vi "Collision Detection top level.vi"(0 "Model rotation (absolute, degrees)":sgl, 1 "Model rotation axis (unit vector)":sgl[](array[numeric])=[0.0, 0.0, 1.0], 3 "Model rotation axis coordinates (absolute, mm)":sgl[](array[numeric])=[0.0, 0.0, 0.0], 4 "Collision mode":T1=enum."Traverse - All", 5 "Get minimum separation within look-out sphere":bool, 6 "Traverse position (absolute, mm)":sgl[](array[numeric])=[0.0, 0.0, 0.0], 7 "3D graphics output":bool, 9 "Visualisation only (no collision detection)":bool, 10 "Traverse name":string, 11 "Extrusion mode":bool, 12 "Rig geometry directory path":path, 13 "Traverse extruded position":sgl[](array[numeric])=[0.0, 0.0, 0.0]) -> (14 "Collision":bool, 15 "Collision point(s)":sgl[][](array[numeric]), 17 "Minimum separation":sgl, 18 "Minimum separation vector (from trav.)":sgl[](array[numeric]), 19 "Error out":errorcluster)   [LabVIEW 2014]
uses:
  Collision Mode.ctl
  Typedefs/Triangle.ctl
  <vilib>/Utility/miscctls.llb/LVRGBAColorTypeDef.ctl
  Collision Detection global.vi
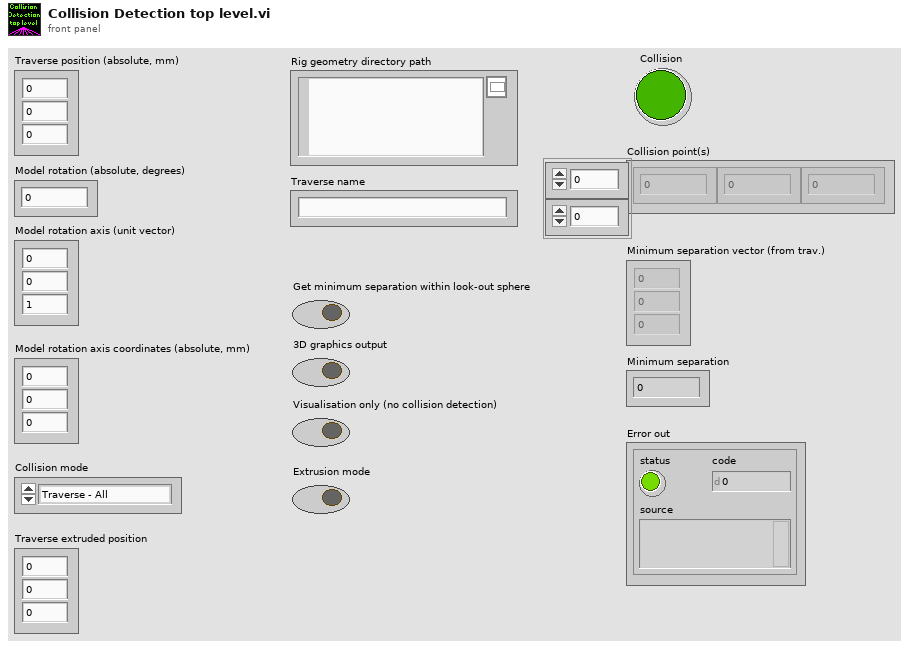
[diagram p1: front panel]
types:
  T1 = typedef "Collision Mode.ctl" = enum16{"Traverse - Tunnel", "Traverse - Model", "Traverse - Traverse", "Traverse - All"}
  T2 = typedef "LVRGBAColorTypeDef.ctl" = cluster{"Red":sgl, "Green":sgl, "Blue":sgl, "Alpha":sgl}
  T3 = cluster{"Red":sgl, "Green":sgl, "Blue":sgl, "Alpha":sgl}
  T4 = typedef "TreeNodeBox.ctl" = cluster{"Face 0":T5, "Face 1":T5, "Face 2":T5, "Face 3":T5, "Face 4":T5, "Face 5":T5, "Level":i32, "Pmax":sgl[], "Pmin":sgl[], "Parent":i32, "Child 1":i32, "Child 2":i32, "Child 3":i32, "Child 4":i32, "Child 5":i32, "Child 6":i32, "Child 7":i32, "Child 8":i32, "Triangles":i32[], "is leaf node":bool}
  T5 = typedef "Quad.ctl" = cluster{"V0":sgl[], "V1":sgl[], "V2":sgl[], "V3":sgl[], "E0":sgl[], "E1":sgl[], "E2":sgl[], "E3":sgl[], "n^":sgl[], "nE0^":sgl[], "nE1^":sgl[], "nE2^":sgl[], "nE3^":sgl[]}
  T6 = typedef "Triangle.ctl" = cluster{"V0":sgl[], "V1":sgl[], "V2":sgl[], "E0":sgl[], "E1":sgl[], "E2":sgl[], "n^":sgl[], "nE0^":sgl[], "nE1^":sgl[], "nE2^":sgl[]}
  T7 = typedef "Sphere.ctl" = cluster{"Centre":sgl[], "Radius":sgl}
  T8 = enum16{"Inherit Value", "Points", "Wireframe", "Polygons"}
  T9 = typedef "LV3DPointTypeDef.ctl" = cluster{"X":sgl, "Y":sgl, "Z":sgl}
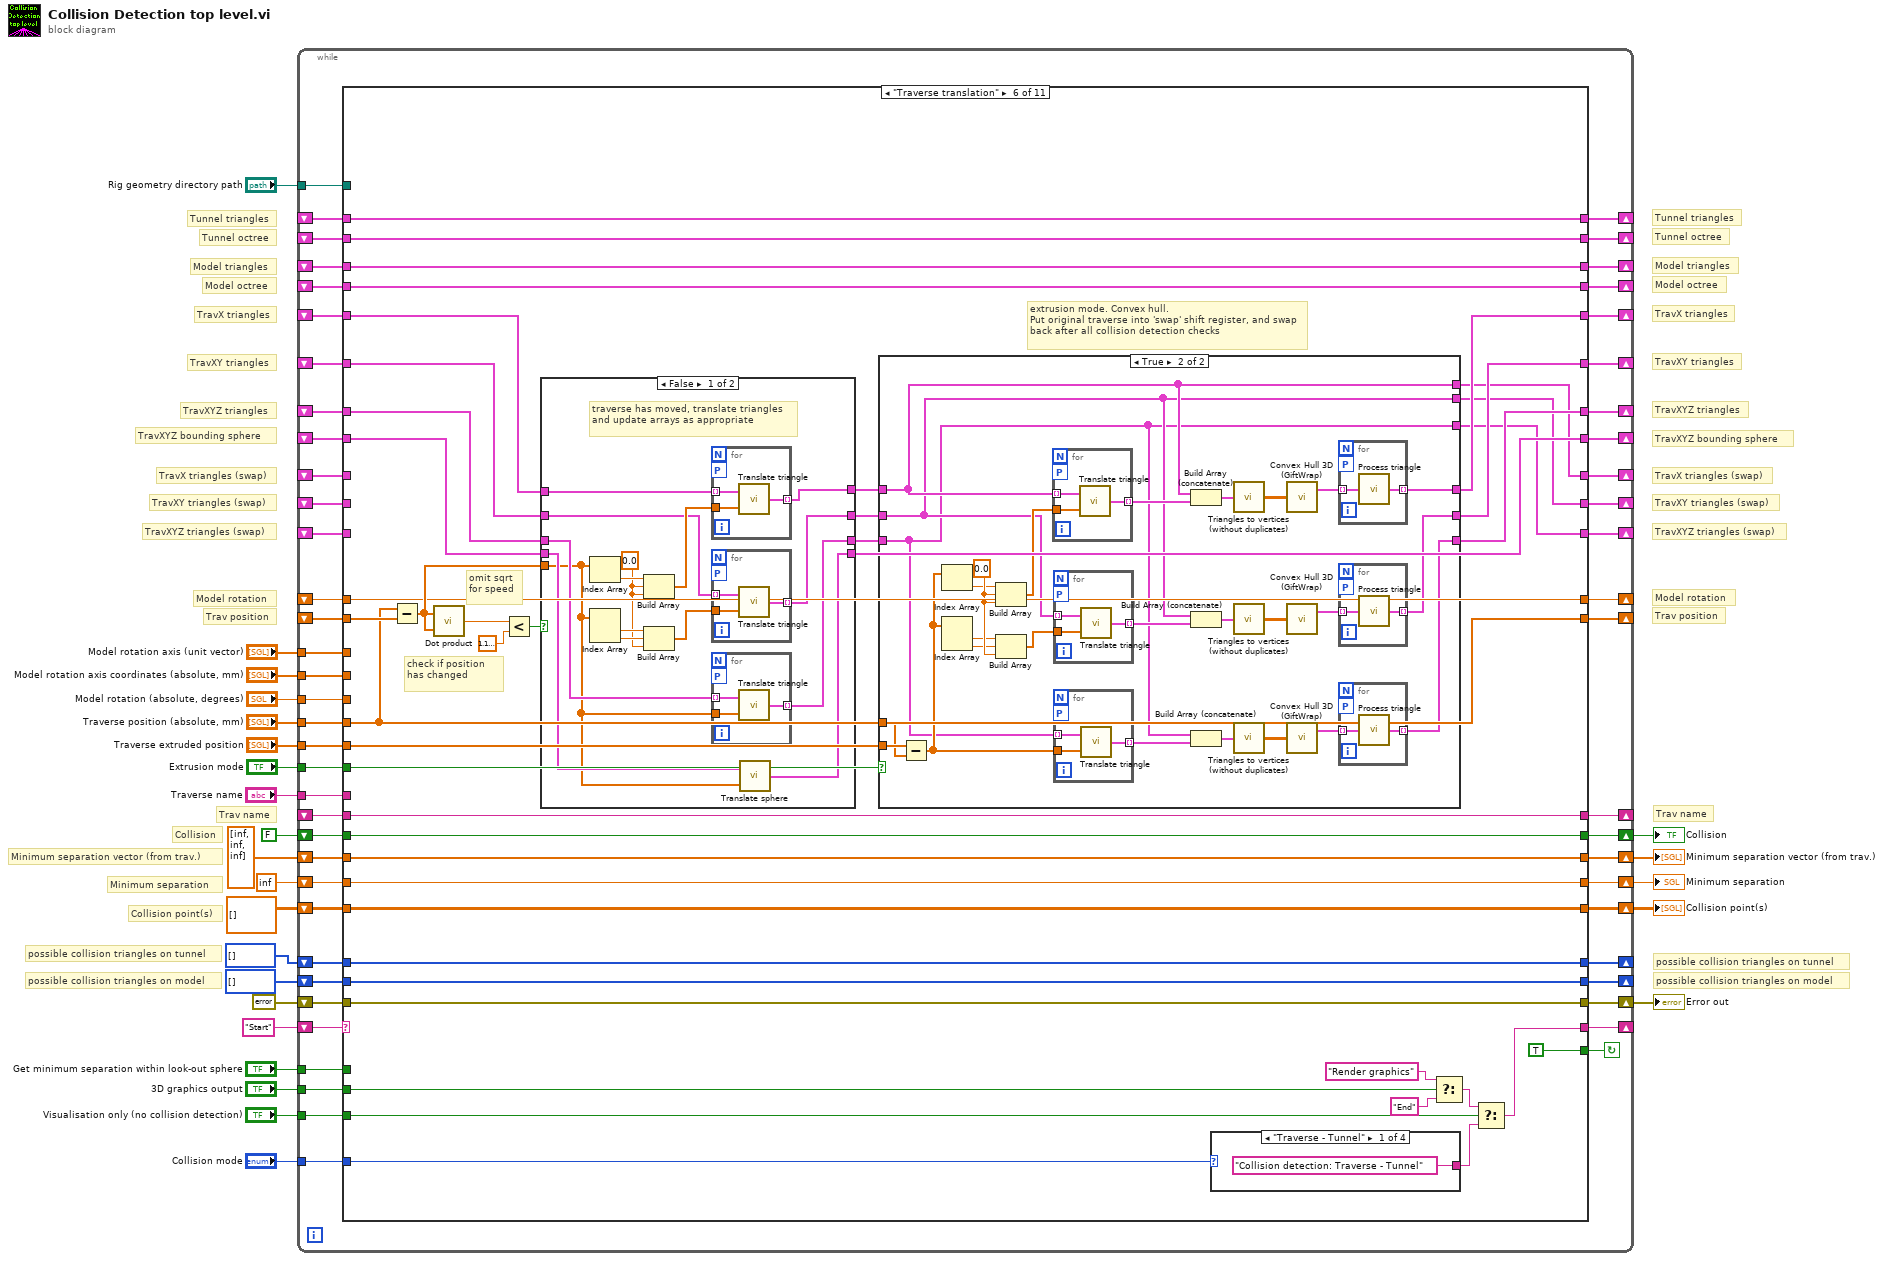
[diagram p0: block diagram]
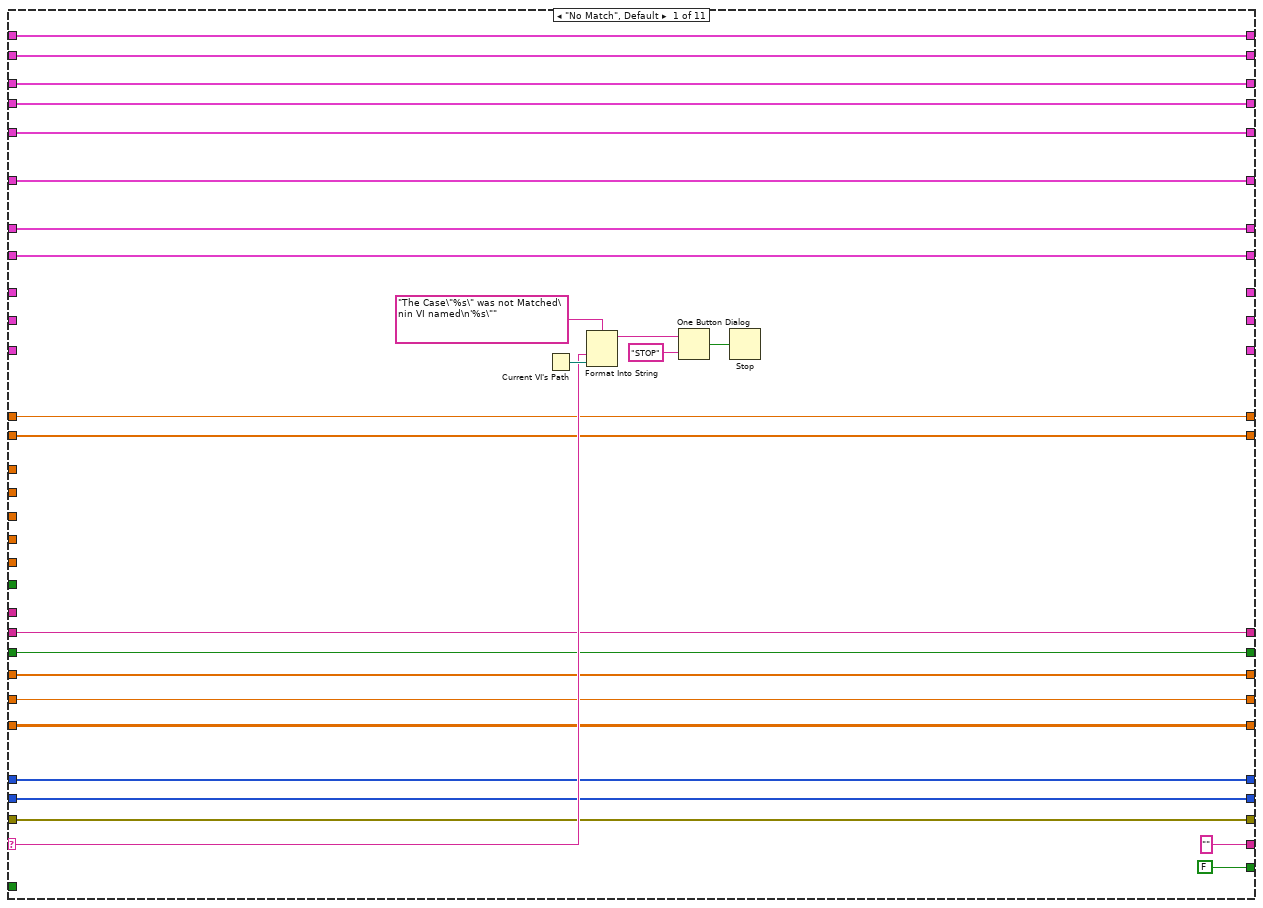
[diagram p2: hidden frame]
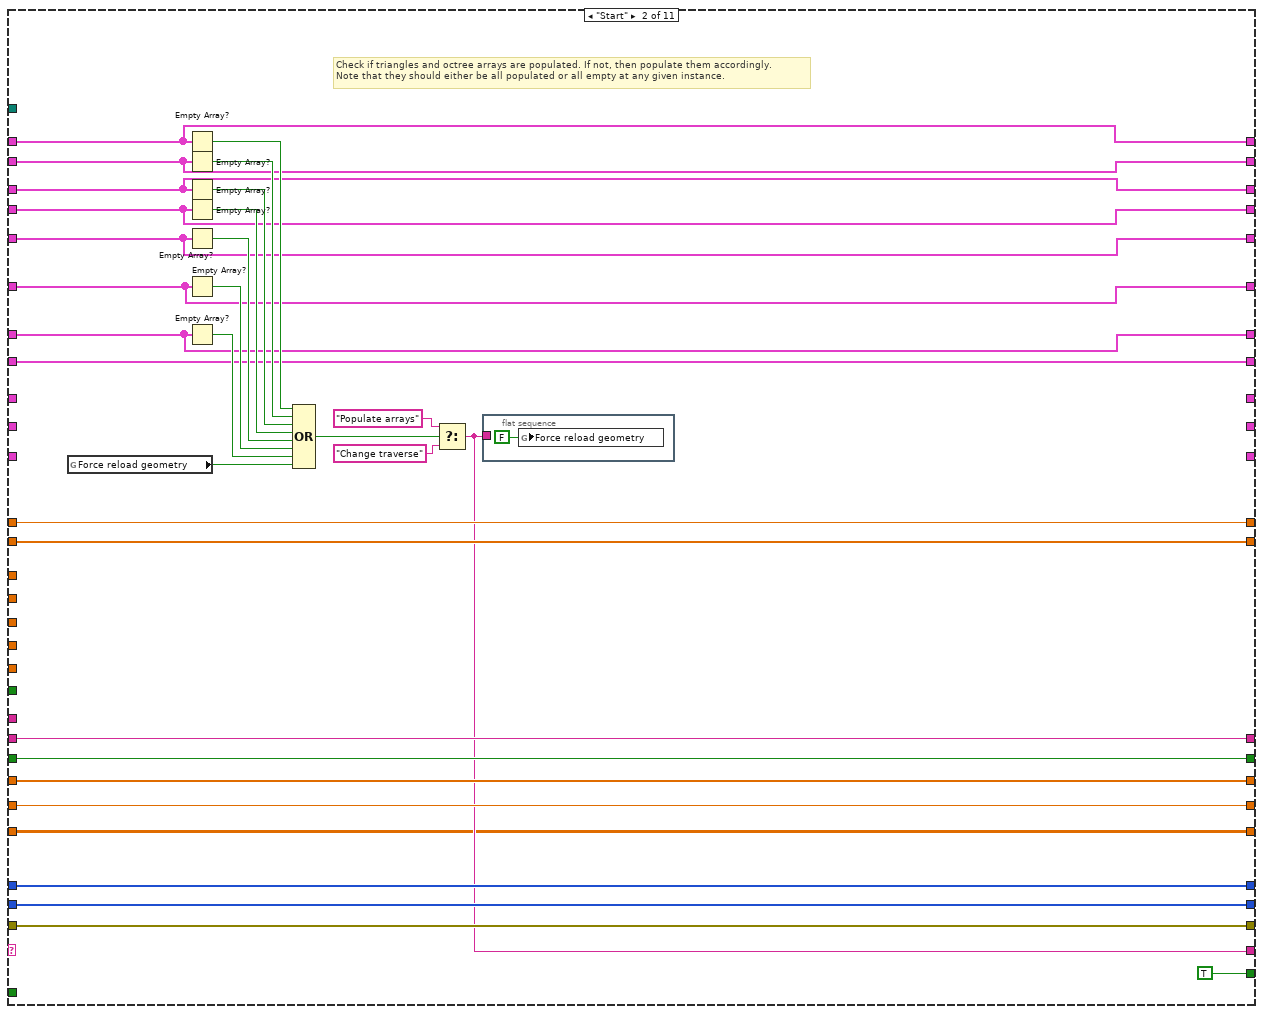
[diagram p3: hidden frame]
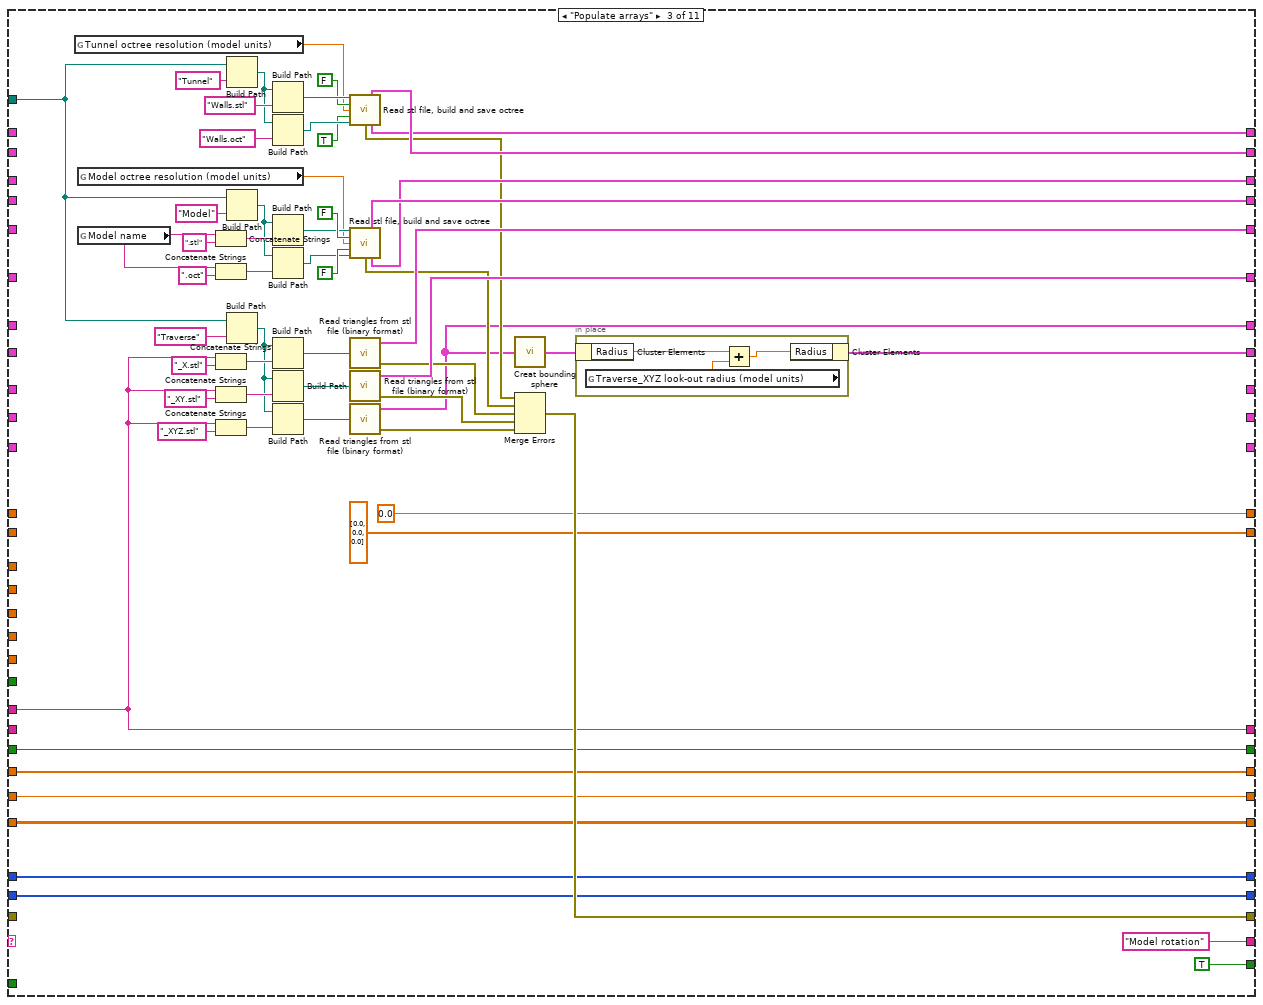
[diagram p4: hidden frame]
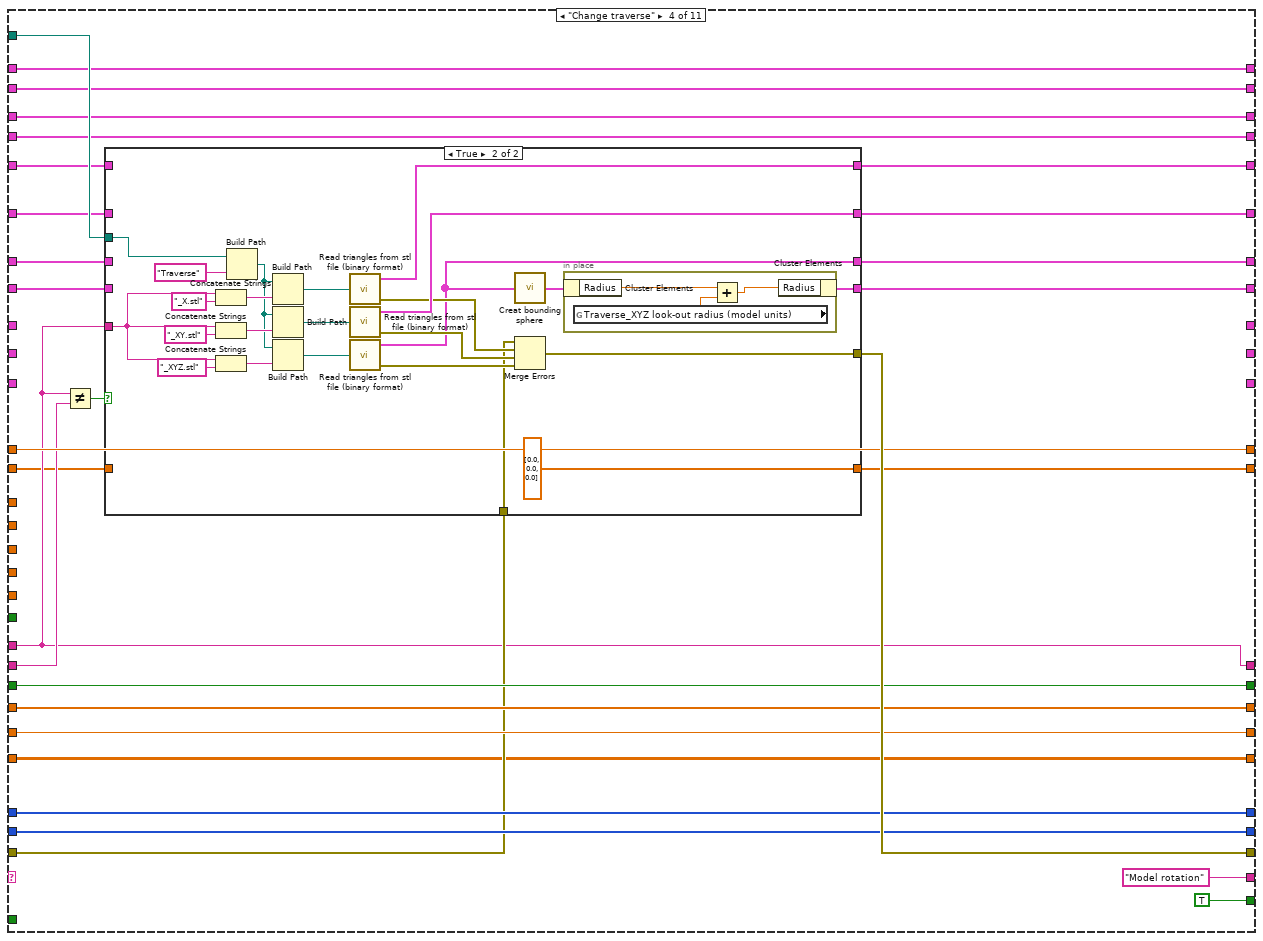
[diagram p5: hidden frame]
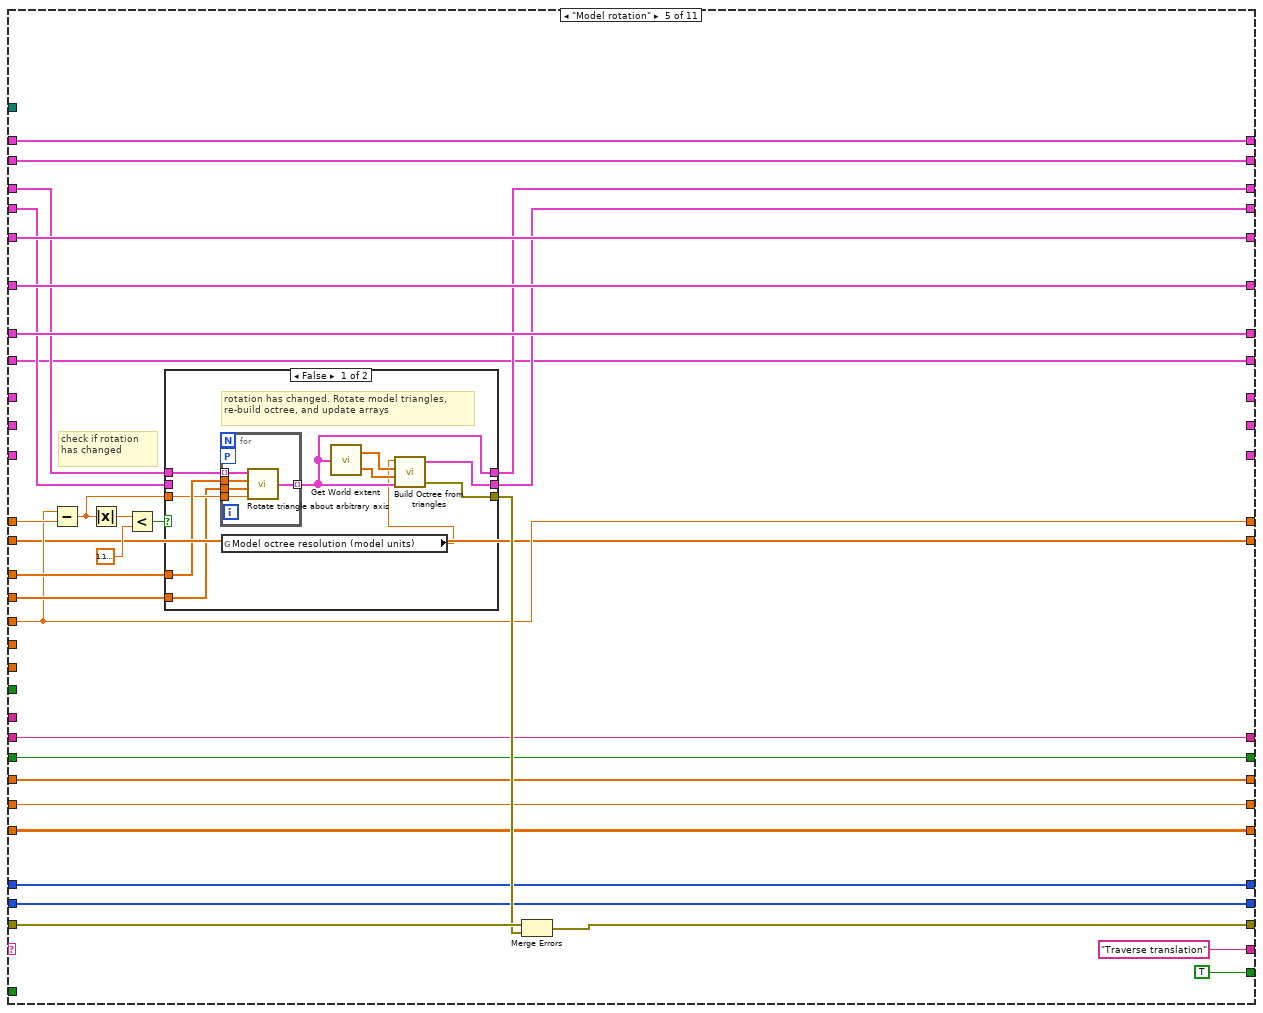
[diagram p7: hidden frame]
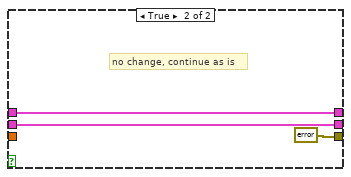
[diagram p8: hidden frame]
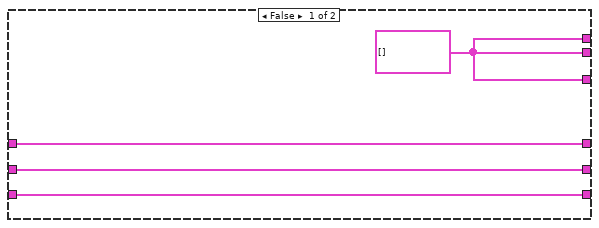
[diagram p9: hidden frame]
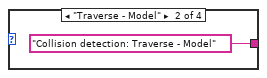
[diagram p10: hidden frame]
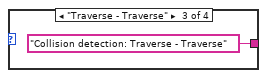
[diagram p11: hidden frame]
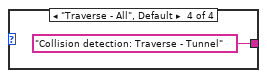
[diagram p12: hidden frame]
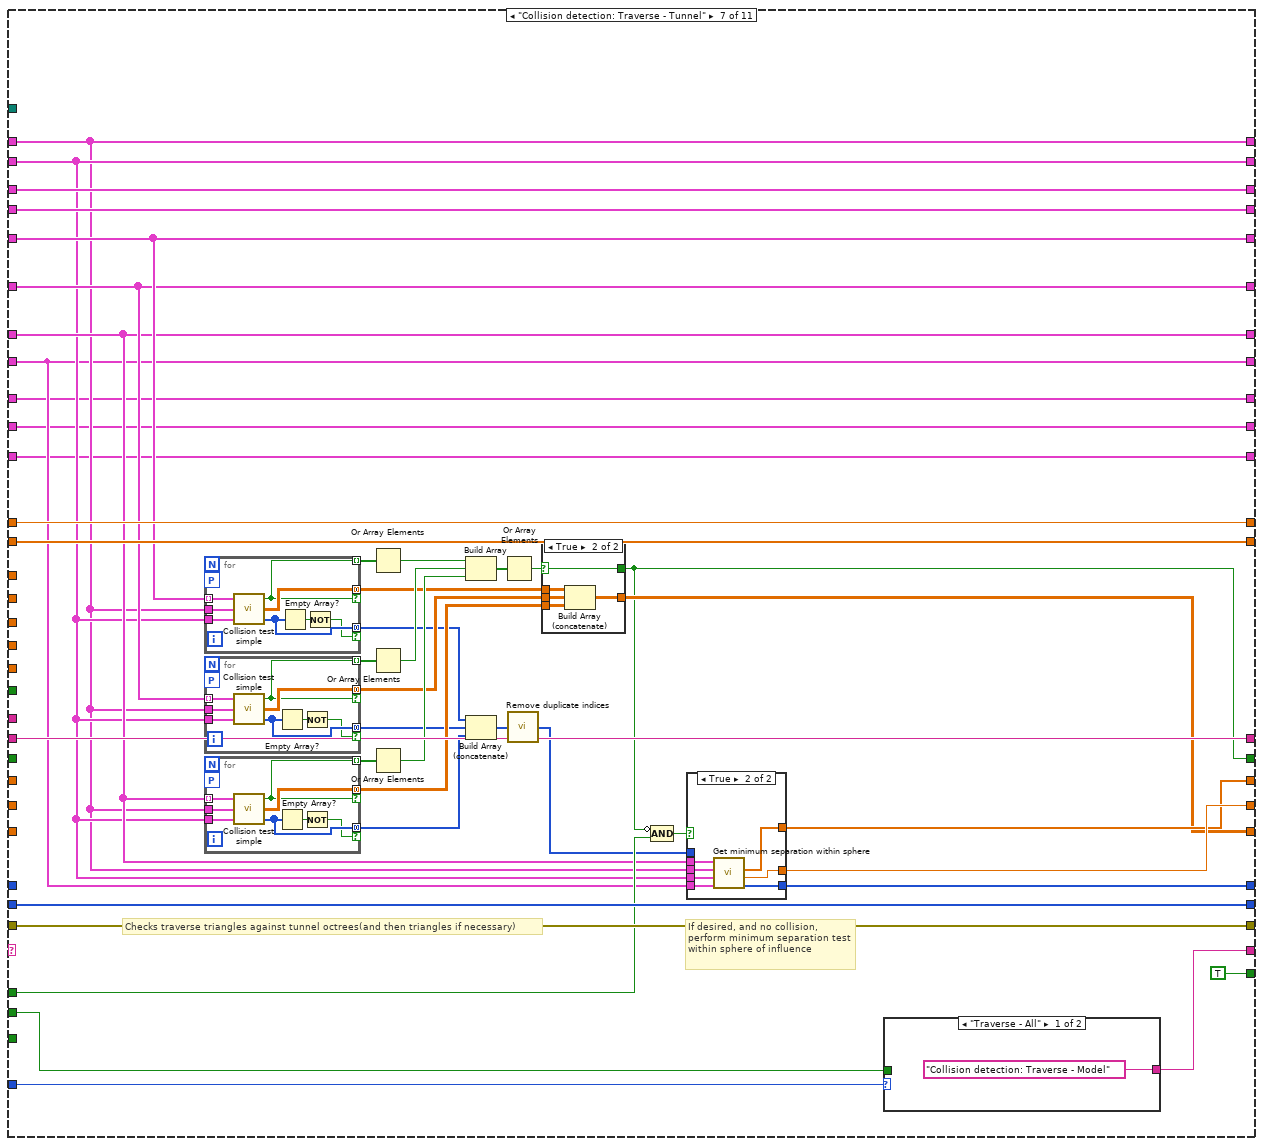
[diagram p14: hidden frame]
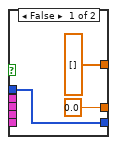
[diagram p15: hidden frame]
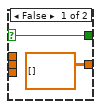
[diagram p16: hidden frame]
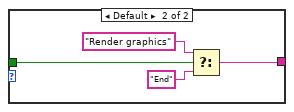
[diagram p17: hidden frame]
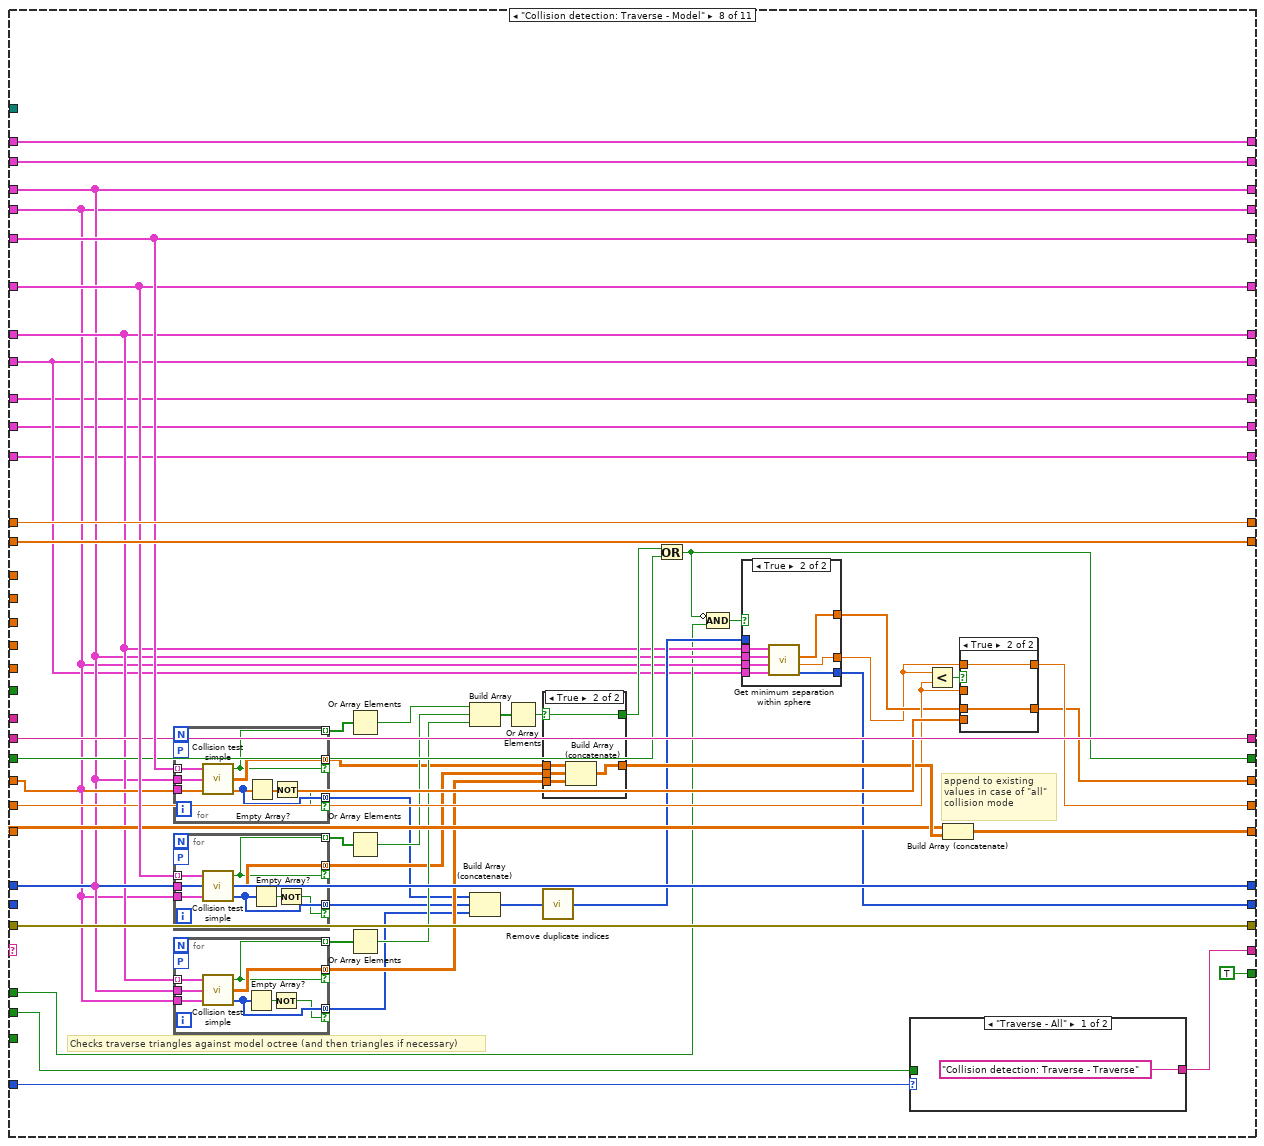
[diagram p18: hidden frame]
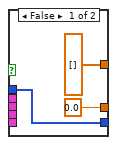
[diagram p19: hidden frame]
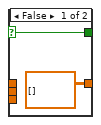
[diagram p20: hidden frame]
diagram:
  # "TravXYZ triangles (swap)"
  # "TravXY triangles (swap)"
  # "TravX triangles (swap)"
  # "TravXYZ triangles (swap)"
  # "TravXY triangles (swap)"
  # "TravX triangles (swap)"
  # "TravXYZ bounding sphere"
  # "TravXYZ bounding sphere"
  # "Trav name"
  # "Collision"
  # "Minimum separation vector (from trav.)"
  # "Minimum separation"
  # "Collision point(s)"
  # "Trav name"
  # "possible collision triangles on tunnel"
  # "possible collision triangles on model"
  # "possible collision triangles on tunnel"
  # "possible collision triangles on model"
  # "Model rotation"
  # "Trav position"
  # "TravXYZ triangles"
  # "TravXY triangles"
  # "TravX triangles"
  # "Model octree"
  # "Model triangles"
  # "Tunnel octree"
  # "Tunnel triangles"
  # "Model rotation"
  # "Trav position"
  # "TravXYZ triangles"
  # "TravXY triangles"
  # "TravX triangles"
  # "Model octree"
  # "Model triangles"
  # "Tunnel octree"
  # "Tunnel triangles"
  n1 = while {
    shift-right: [w64] -> _
    shift-left: "Start" -> [w82]
    shift-right: [w71] -> _
    shift-left: _ -> [w81]
    shift-right: [w70] -> _
    shift-left: _ -> [w80]
    shift-right: [w69] -> _
    shift-left: _ -> [w79]
    shift-right: [w68] -> _
    shift-left: _ -> [w78]
    shift-right: [w67] -> _
    shift-left: _ -> [w77]
    shift-right: [w66] -> _
    shift-left: _ -> [w76]
    shift-right: [w65] -> _
    shift-left: _ -> [w54]
    shift-right: [w58] -> _
    shift-left: _ -> [w74]
    shift-right: [w57] -> _
    shift-left: _ -> [w75]
    tunnel: "Traverse position (absolute, mm)" -> [w72]
    tunnel: "Model rotation (absolute, degrees)" -> [w73]
    tunnel: "Rig geometry directory path" -> [w62]
    shift-right: [w60] -> w12
    shift-left: errorcluster {"status"=FALSE, "code"=0, "source"=""} ("error IO") -> [w59]
    tunnel: "Model rotation axis (unit vector)" -> [w56]
    tunnel: "Model rotation axis coordinates (absolute, mm)" -> [w55]
    tunnel: "Get minimum separation within look-out sphere" -> [w53]
    tunnel: "Visualisation only (no collision detection)" -> [w52]
    tunnel: "3D graphics output" -> [w51]
    shift-right: [w47] -> _
    shift-left: i32[] [] ("I32 array without duplicates") -> [w45]
    shift-right: [w46] -> _
    shift-left: i32[] [] ("I32 array without duplicates") -> [w44]
    shift-right: [w48] -> w14
    shift-left: sgl[] [inf, inf, inf] -> [w43]
    shift-right: [w49] -> w15
    shift-left: sgl inf -> [w42]
    shift-right: [w36] -> w13
    shift-left: sgl[][] [] -> [w41]
    shift-right: [w50] -> w16
    shift-left: FALSE -> [w40]
    shift-right: [w39] -> _
    shift-left: _ -> [w61]
    tunnel: "Traverse name" -> [w38]
    tunnel: "Collision mode" -> [w37]
    shift-right: [w34] -> _
    shift-left: _ -> [w35]
    tunnel: "Traverse extruded position" -> [w33]
    tunnel: "Extrusion mode" -> [w32]
    shift-right: [w31] -> _
    shift-left: _ -> [w28]
    shift-right: [w30] -> _
    shift-left: _ -> [w27]
    shift-right: [w29] -> _
    shift-left: _ -> [w26]
    stop <- w63 continue-if-true
    n2 = case shown="\"Traverse translation\"" w82 {
      selector: w82 -> [w103 _ _ _ _ _ _ _ _ _ _]
      tunnel: w81 -> [w99 w121 _ w218 w291 w350 w440 w571 w643 w710 w825]
      tunnel: w80 -> [w98 w122 _ w217 w290 w349 w441 w570 w642 w706 w824]
      tunnel: w79 -> [w97 w123 _ w216 w286 w348 w472 w531 w639 w666 w823]
      tunnel: w78 -> [w96 w124 _ w215 w279 w347 w471 w530 w638 w705 w822]
      tunnel: w77 -> [w95 w125 _ w211 w289 w354 w474 w572 w644 w709 w804]
      tunnel: w76 -> [w94 w126 _ w210 w288 w353 w473 w569 w641 w708 w805]
      tunnel: w54 -> [w93 w127 _ w209 w287 w352 w442 w532 w640 w707 w806]
      tunnel: w75 -> [w91 w119 _ w207 w267 w357 w477 w575 w651 w714 w827]
      tunnel: w74 -> [w92 w120 _ w224 w284 w331 w478 w576 w652 w715 w826]
      tunnel: w73 -> [_ _ _ _ w274 _ _ _ _ _ _]
      tunnel: w72 -> [_ _ _ _ _ w323 _ _ _ _ _]
      tunnel: [w99 w121 w194 w218 w291 w350 w440 w571 w643 w710 w825] -> w71
      tunnel: [w98 w122 w195 w217 w290 w349 w441 w570 w642 w706 w824] -> w70
      tunnel: [w97 w123 w196 w216 w281 w348 w472 w531 w639 w666 w823] -> w69
      tunnel: [w96 w124 w197 w215 w280 w347 w471 w530 w638 w705 w822] -> w68
      tunnel: [w95 w125 w198 w229 w289 w319 w474 w572 w644 w709 w809] -> w67
      tunnel: [w94 w126 w199 w230 w288 w318 w473 w569 w641 w708 w808] -> w66
      tunnel: [w93 w127 w143 w231 w287 w317 w442 w532 w640 w707 w807] -> w65
      tunnel: [w92 w120 sgl 0.0 ("Numeric") w224 w274 w331 w478 w576 w652 w715 w826] -> w58
      tunnel: [w91 w119 sgl[] [0.0, 0.0, 0.0] ("Traverse position (absolute, mm)") w206 w267 w323 w477 w575 w651 w714 w827] -> w57
      tunnel: w62 -> [_ _ w193 w228 _ _ _ _ _ _ _]
      tunnel: ["" w111 "Model rotation" "Model rotation" "Traverse translation" w343 w463 w560 w647 "End" "" ("f")] -> w64
      tunnel: [FALSE TRUE TRUE TRUE TRUE TRUE TRUE TRUE TRUE TRUE FALSE] -> w63
      tunnel: w61 -> [w85 w113 _ w213 w268 w333 w468 w568 w637 w675 w816]
      tunnel: [w100 w128 w192 w227 w278 w345 w475 w573 w645 w693 w828] -> w60
      tunnel: w59 -> [w100 w128 _ w214 w277 w345 w475 w573 w645 w694 w828]
      tunnel: w56 -> [_ _ _ _ w292 _ _ _ _ _ _]
      tunnel: w55 -> [_ _ _ _ w282 _ _ _ _ _ _]
      tunnel: w53 -> [_ _ _ _ _ _ w446 w529 _ _ _]
      tunnel: w52 -> [_ _ _ _ _ w344 _ _ _ _ _]
      tunnel: w51 -> [_ _ _ _ _ w342 w464 w559 w648 _ _]
      tunnel: [w86 w114 w152 w219 w269 w334 w447 w533 w636 w711 w817] -> w50
      tunnel: [w87 w115 w153 w220 w270 w335 w470 w564 w634 w712 w818] -> w49
      tunnel: [w88 w116 w154 w221 w271 w336 w469 w563 w635 w713 w819] -> w48
      tunnel: [w84 w110 w144 w205 w266 w328 w466 w566 w631 w658 w815] -> w36
      tunnel: [w90 w117 w155 w222 w272 w337 w443 w567 w633 w685 w820] -> w47
      tunnel: [w89 w118 w156 w223 w273 w338 w467 w534 w632 w664 w821] -> w46
      tunnel: w45 -> [w90 w117 w155 w222 w272 w337 _ w567 w633 w685 w820]
      tunnel: w44 -> [w89 w118 w156 w223 w273 w338 w467 _ w632 w664 w821]
      tunnel: w43 -> [w88 w116 w154 w221 w271 w336 _ w562 w635 w713 w819]
      tunnel: w42 -> [w87 w115 w153 w220 w270 w335 _ w554 w634 w712 w818]
      tunnel: w41 -> [w84 w110 w144 w205 w266 w328 _ w555 w631 w658 w815]
      tunnel: w40 -> [w86 w114 w152 w219 w269 w334 _ w557 w636 w711 w817]
      tunnel: [w85 w113 w151 w208 w268 w333 w468 w568 w637 w675 w816] -> w39
      tunnel: w38 -> [_ _ w151 w208 _ _ _ _ _ _ _]
      tunnel: w37 -> [_ _ _ _ _ w330 w465 w561 _ _ _]
      tunnel: w35 -> [w83 w109 _ w203 w265 w327 w439 w528 w630 w657 w814]
      tunnel: [w83 w109 w141 w204 w265 w326 w439 w528 w630 w657 w814] -> w34
      tunnel: w33 -> [_ _ _ _ _ w324 _ _ _ _ _]
      tunnel: w32 -> [_ _ _ _ _ w325 _ _ _ _ w813]
      tunnel: [_ _ _ _ _ w314 w438 w527 w629 w656 _] -> w31
      tunnel: [_ _ _ _ _ w315 w437 w526 w628 w655 _] -> w30
      tunnel: [_ _ _ _ _ w316 w436 w525 w627 w654 _] -> w29
      tunnel: w28 -> [_ _ _ _ _ _ w438 w527 w629 w656 w812]
      tunnel: w27 -> [_ _ _ _ _ _ w437 w526 w628 w655 w811]
      tunnel: w26 -> [_ _ _ _ _ _ w436 w525 w627 w654 w810]
      frame "No Match", Default {
        n3 = Current VI's Path() -> (path=w104:path)
        n4 = Format Into String(format string="The Case\"%s\" was not Matched\nin VI named\n'%s\"" ("Format String"), w103, w104) -> (resulting string=w107:string)  [unwired: 2 in, 1 out]
        n5 = One Button Dialog(message=w107, button name ("OK")="STOP") -> (true=w105:bool)
        n6 = Stop(stop? (T)=w105) -> ()
      }
      frame "Start" {
        # "Check if triangles and octree arrays are populated. If not, then populate them accordingly.\nNote that they should either be all populated or all empty at any given instance."
        n7 = global read "Collision Detection global.vi" "Force reload geometry"() -> (w112:bool)
        n8 = Empty Array?(array=w121) -> (empty?=w139:bool)
        n9 = Empty Array?(array=w122) -> (empty?=w138:bool)
        n10 = Empty Array?(array=w123) -> (empty?=w137:bool)
        n11 = Empty Array?(array=w124) -> (empty?=w136:bool)
        n12 = Empty Array?(array=w125) -> (empty?=w135:bool)
        n13 = Empty Array?(array=w126) -> (empty?=w134:bool)
        n14 = Empty Array?(array=w127) -> (empty?=w133:bool)
        n15 = Compound Arithmetic op=OR(w139, w138, w137, w136, w135, w134, w133, w112) -> (w132:bool)
        n16 = Select(t="Populate arrays", s=w132, f="Change traverse") -> (s? t:f=w111:string)
        n17 = flat-sequence {
          tunnel: w111 -> [_]
          frame #0 {
            n18 = global write "Collision Detection global.vi" "Force reload geometry"(FALSE ("Force reload geometry")) -> ()
          }
        }
      }
      frame "Populate arrays" {
        n19 = global read "Collision Detection global.vi" "Tunnel octree resolution (model units)"() -> (w149:sgl)
        n20 = global read "Collision Detection global.vi" "Model octree resolution (model units)"() -> (w148:sgl)
        n21 = global read "Collision Detection global.vi" "Model name"() -> (w147:string)
        n22 = Concatenate Strings(w147, ".stl" ("string")) -> (w180:string)
        n23 = Concatenate Strings(w147, ".oct" ("string")) -> (w179:string)
        n24 = Concatenate Strings(w151, "_X.stl" ("string")) -> (w173:string)
        n25 = Concatenate Strings(w151, "_XY.stl" ("string")) -> (w164:string)
        n26 = Concatenate Strings(w151, "_XYZ.stl" ("string")) -> (w162:string)
        n27 = Build Path(base path=w193, name or relative path="Tunnel") -> (appended path=w188:path)
        n28 = Build Path(base path=w193, name or relative path="Model") -> (appended path=w178:path)
        n29 = Build Path(base path=w193, name or relative path="Traverse") -> (appended path=w150:path)
        n30 = Build Path(base path=w188, name or relative path="Walls.stl") -> (appended path=w189:path)
        n31 = Build Path(base path=w188, name or relative path="Walls.oct") -> (appended path=w186:path)
        n32 = Build Path(base path=w178, name or relative path=w180) -> (appended path=w175:path)
        n33 = Build Path(base path=w178, name or relative path=w179) -> (appended path=w174:path)
        n34 = Build Path(base path=w150, name or relative path=w173) -> (appended path=w170:path)
        n35 = Build Path(base path=w150, name or relative path=w164) -> (appended path=w166:path)
        n36 = Build Path(base path=w150, name or relative path=w162) -> (appended path=w160:path)
        n37 = call "Read stl file, build and save octree.vi"("STL file path (load)"=w189, "Auto resolution"=FALSE, "Specify resolution"=w149, "Invert model (interior region)"=TRUE, "Octree file path (save)"=w186) -> ("Octree node array"=w195:T4[], "Error out"=w169:errorcluster, "Triangles array"=w194:T6[])  [unwired: 3 in, 5 out]
        n38 = call "Read stl file, build and save octree.vi"("STL file path (load)"=w175, "Auto resolution"=FALSE, "Specify resolution"=w148, "Invert model (interior region)"=FALSE, "Octree file path (save)"=w174) -> ("Octree node array"=w197:T4[], "Error out"=w168:errorcluster, "Triangles array"=w196:T6[])  [unwired: 3 in, 5 out]
        n39 = call "Read triangles from stl file (binary format).vi"("STL file path"=w170) -> ("Triangles array"=w198:T6[], "Error out"=w167:errorcluster)  [unwired: 1 out]
        n40 = call "Read triangles from stl file (binary format).vi"("STL file path"=w166) -> ("Triangles array"=w199:T6[], "Error out"=w163:errorcluster)  [unwired: 1 out]
        n41 = call "Read triangles from stl file (binary format).vi"("STL file path"=w160) -> ("Triangles array"=w143:T6[], "Error out"=w159:errorcluster)  [unwired: 1 out]
        n42 = call "Creat bounding sphere.vi"("Triangles"=w143) -> ("Bounding sphere"=w142:T7)
        n43 = Merge Errors(w169, w168, w167, w163, w159) -> (w192:errorcluster)
        n44 = in-place {
          n45 = in-place-cluster #1(w142) -> ("Radius"=w202:sgl)
          n46 = global read "Collision Detection global.vi" "Traverse_XYZ look-out radius (model units)"() -> (w201:sgl)
          n47 = Add(x=w202, y=w201) -> (x+y=w200:sgl)
          n48 = in-place-cluster #1("Radius"=w200) -> (w141:T7)
        }
      }
      frame "Change traverse" {
        n49 = Not Equal?(x=w208, y=w213) -> (x != y?=w212:bool)
        n50 = case shown="True" w212 {
          tunnel: [w235 w240] -> w231
          tunnel: [w236 w261] -> w230
          tunnel: [w237 w260] -> w229
          tunnel: w228 -> [_ w259]
          tunnel: [w234 w258] -> w227
          tunnel: w208 -> [_ w242]
          tunnel: w214 -> [w234 w244]
          tunnel: w211 -> [w237 _]
          tunnel: w210 -> [w236 _]
          tunnel: w209 -> [w235 _]
          tunnel: w207 -> [w233 _]
          tunnel: [w233 sgl[] [0.0, 0.0, 0.0] ("Traverse position (absolute, mm)")] -> w206
          tunnel: [w232 w238] -> w204
          tunnel: w203 -> [w232 _]
          frame False {
          }
          frame True {
            n51 = Concatenate Strings(w242, "_X.stl" ("string")) -> (w257:string)
            n52 = Concatenate Strings(w242, "_XY.stl" ("string")) -> (w250:string)
            n53 = Concatenate Strings(w242, "_XYZ.stl" ("string")) -> (w248:string)
            n54 = Build Path(base path=w259, name or relative path="Traverse") -> (appended path=w243:path)
            n55 = Build Path(base path=w243, name or relative path=w257) -> (appended path=w254:path)
            n56 = Build Path(base path=w243, name or relative path=w250) -> (appended path=w252:path)
            n57 = Build Path(base path=w243, name or relative path=w248) -> (appended path=w246:path)
            n58 = call "Read triangles from stl file (binary format).vi"("STL file path"=w254) -> ("Triangles array"=w260:T6[], "Error out"=w253:errorcluster)  [unwired: 1 out]
            n59 = call "Read triangles from stl file (binary format).vi"("STL file path"=w252) -> ("Triangles array"=w261:T6[], "Error out"=w249:errorcluster)  [unwired: 1 out]
            n60 = call "Read triangles from stl file (binary format).vi"("STL file path"=w246) -> ("Triangles array"=w240:T6[], "Error out"=w245:errorcluster)  [unwired: 1 out]
            n61 = call "Creat bounding sphere.vi"("Triangles"=w240) -> ("Bounding sphere"=w239:T7)
            n62 = Merge Errors(w244, w253, w249, w245) -> (w258:errorcluster)
            n63 = in-place {
              n64 = in-place-cluster #2(w239) -> ("Radius"=w264:sgl)
              n65 = global read "Collision Detection global.vi" "Traverse_XYZ look-out radius (model units)"() -> (w263:sgl)
              n66 = Add(x=w264, y=w263) -> (x+y=w262:sgl)
              n67 = in-place-cluster #2("Radius"=w262) -> (w238:T7)
            }
          }
        }
      }
      frame "Model rotation" {
        # "check if rotation has changed"
        n68 = Subtract(x=w274, y=w284) -> (x-y=w285:sgl)
        n69 = Absolute Value(x=w285) -> (abs(x)=w295:sgl)
        n70 = Less?(x=w295, y=sgl 1.1920929e-07) -> (x < y?=w293:bool)
        n71 = case shown="False" w293 {
          tunnel: w292 -> [w304 _]
          tunnel: w286 -> [w305 w311]
          tunnel: w285 -> [w303 _]
          tunnel: w282 -> [w302 _]
          tunnel: [w299 w311] -> w281
          tunnel: [w298 w312] -> w280
          tunnel: [w297 errorcluster {"status"=FALSE, "code"=0, "source"=""} ("Stack error")] -> w276
          tunnel: w279 -> [_ w312]
          frame False {
            # "rotation has changed. Rotate model triangles, re-build octree, and update arrays"
            n72 = for {
              tunnel: w305 -> [w310] mode=indexing
              tunnel: w304 -> [w309]
              tunnel: w303 -> [w308]
              tunnel: [w306] -> w299 mode=indexing
              tunnel: w302 -> [w307]
              workers-P: _ -> [_]
              n73 = call "Rotate triangle about arbitrary axis.vi"("Rotation angle (rad)"=w308, "Rotation axis coordinates (x, y, z)"=w307, "Rotation axis (unit direction vector)\nanti-clockwise positive looking into axis"=w309, "Triangle in"=w310) -> ("Triangle out"=w306:T6)
            }
            n74 = global read "Collision Detection global.vi" "Model octree resolution (model units)"() -> (w296:sgl)
            n75 = call "Get World extent.vi"("Triangles"=w299) -> ("Pmax (x, y, z)"=w300:sgl[], "Pmin (x, y, z)"=w301:sgl[])
            n76 = call "Build Octree from triangles.vi"("Triangle array"=w299, "World Pmin (x, y, z)"=w301, "World Pmax (x, y, z)"=w300, "Octree resolution (model units)"=w296) -> ("Stack error"=w297:errorcluster, "Octree node array"=w298:T4[])  [unwired: 1 out]
          }
          frame True {
            # "no change, continue as is"
          }
        }
        n77 = Merge Errors(w277, w276) -> (w278:errorcluster)
      }
      frame "Traverse translation" {
        # "extrusion mode. Convex hull.\nPut original traverse into 'swap' shift register, and swap back after all collision detection checks"
        # "omit sqrt for speed"
        # "check if position has changed"
        n78 = Subtract(x=w323, y=w357) -> (x-y=w351:sgl[])
        n79 = call "Dot product.vi"("B"=w351, "A"=w351) -> ("A . B"=w332:sgl)
        n80 = Less?(x=w332, y=sgl 1.1920929e-07) -> (x < y?=w355:bool)
        n81 = case shown="False" w355 {
          tunnel: w354 -> [w422 w435]
          tunnel: w353 -> [w416 w434]
          tunnel: w352 -> [w414 w433]
          tunnel: w351 -> [w409 _]
          tunnel: [w413 w435] -> w322
          tunnel: [w412 w434] -> w321
          tunnel: [w411 w433] -> w320
          tunnel: w327 -> [w410 w432]
          tunnel: [w408 w432] -> w326
          frame False {
            w418 = sgl 0.0 ("element")
            # "traverse has moved, translate triangles and update arrays as appropriate"
            n82 = Index Array(array=w409) -> (element=w421:sgl)  [unwired: 1 in]
            n83 = Index Array(array=w409) -> (element #1=w419:sgl, element #2=w420:sgl)  [unwired: 2 in]
            n84 = Build Array(w421, w418, w418) -> (w417:sgl[])
            n85 = Build Array(w419, w420, w418) -> (w415:sgl[])
            n86 = for {
              tunnel: w422 -> [w431] mode=indexing
              workers-P: _ -> [_]
              tunnel: w417 -> [w430]
              tunnel: [w429] -> w413 mode=indexing
              n87 = call "Translate triangle.vi"("Translation vector (dx, dy, dz)"=w430, "Triangle in"=w431) -> ("Triangle out"=w429:T6)
            }
            n88 = for {
              tunnel: w416 -> [w428] mode=indexing
              workers-P: _ -> [_]
              tunnel: w415 -> [w427]
              tunnel: [w426] -> w412 mode=indexing
              n89 = call "Translate triangle.vi"("Translation vector (dx, dy, dz)"=w427, "Triangle in"=w428) -> ("Triangle out"=w426:T6)
            }
            n90 = for {
              tunnel: w414 -> [w425] mode=indexing
              workers-P: _ -> [_]
              tunnel: w409 -> [w424]
              tunnel: [w423] -> w411 mode=indexing
              n91 = call "Translate triangle.vi"("Translation vector (dx, dy, dz)"=w424, "Triangle in"=w425) -> ("Triangle out"=w423:T6)
            }
            n92 = call "Translate sphere.vi"("Translation vector (dx, dy, dz)"=w409, "Sphere in"=w410) -> ("Sphere out"=w408:T7)
          }
          frame True {
            # "no change, continue as is"
          }
        }
        n93 = case shown="True" w325 {
          tunnel: w320 -> [w359 w362]
          tunnel: [w359 w374] -> w317
          tunnel: w323 -> [_ w387]
          tunnel: w324 -> [_ w388]
          tunnel: w321 -> [w360 w365]
          tunnel: w322 -> [w361 w369]
          tunnel: [w360 w376] -> w318
          tunnel: [w361 w378] -> w319
          tunnel: [w358 w369] -> w314
          tunnel: [w358 w365] -> w315
          tunnel: [w358 w362] -> w316
          frame False {
            w358 = T6[] [] ("Triangles array")
          }
          frame True {
            w386 = sgl 0.0 ("element")
            n94 = Subtract(x=w388, y=w387) -> (x-y=w382:sgl[])
            n95 = Index Array(array=w382) -> (element=w383:sgl)  [unwired: 1 in]
            n96 = Index Array(array=w382) -> (element #1=w385:sgl, element #2=w384:sgl)  [unwired: 2 in]
            n97 = Build Array(w383, w386, w386) -> (w380:sgl[])
            n98 = Build Array(w385, w384, w386) -> (w381:sgl[])
            n99 = for {
              tunnel: w369 -> [w397] mode=indexing
              workers-P: _ -> [_]
              tunnel: w380 -> [w396]
              tunnel: [w395] -> w370 mode=indexing
              n100 = call "Translate triangle.vi"("Translation vector (dx, dy, dz)"=w396, "Triangle in"=w397) -> ("Triangle out"=w395:T6)
            }
            n101 = for {
              tunnel: w365 -> [w400] mode=indexing
              workers-P: _ -> [_]
              tunnel: w381 -> [w399]
              tunnel: [w398] -> w367 mode=indexing
              n102 = call "Translate triangle.vi"("Translation vector (dx, dy, dz)"=w399, "Triangle in"=w400) -> ("Triangle out"=w398:T6)
            }
            n103 = for {
              tunnel: w362 -> [w403] mode=indexing
              workers-P: _ -> [_]
              tunnel: w382 -> [w402]
              tunnel: [w401] -> w364 mode=indexing
              n104 = call "Translate triangle.vi"("Translation vector (dx, dy, dz)"=w402, "Triangle in"=w403) -> ("Triangle out"=w401:T6)
            }
            n105 = Build Array (concatenate)(w369, w370) -> (w368:T6[])
            n106 = Build Array (concatenate)(w365, w367) -> (w366:T6[])
            n107 = Build Array (concatenate)(w362, w364) -> (w363:T6[])
            n108 = call "Triangles to vertices (without duplicates).vi"("Triangles"=w368) -> ("Vertices (without duplicates)"=w371:sgl[][])
            n109 = call "Triangles to vertices (without duplicates).vi"("Triangles"=w366) -> ("Vertices (without duplicates)"=w372:sgl[][])
            n110 = call "Triangles to vertices (without duplicates).vi"("Triangles"=w363) -> ("Vertices (without duplicates)"=w373:sgl[][])
            n111 = call "Convex Hull 3D (GiftWrap).vi"("Vertices"=w371) -> ("Convex hull triangles (partial proc.)"=w379:T6[])  [unwired: 1 out]
            n112 = call "Convex Hull 3D (GiftWrap).vi"("Vertices"=w372) -> ("Convex hull triangles (partial proc.)"=w377:T6[])  [unwired: 1 out]
            n113 = call "Convex Hull 3D (GiftWrap).vi"("Vertices"=w373) -> ("Convex hull triangles (partial proc.)"=w375:T6[])  [unwired: 1 out]
            n114 = for {
              tunnel: w379 -> [w394] mode=indexing
              tunnel: [w393] -> w378 mode=indexing
              workers-P: _ -> [_]
              n115 = call "Process triangle.vi"("Triangle in"=w394) -> ("Triangle out"=w393:T6)
            }
            n116 = for {
              tunnel: w377 -> [w392] mode=indexing
              tunnel: [w391] -> w376 mode=indexing
              workers-P: _ -> [_]
              n117 = call "Process triangle.vi"("Triangle in"=w392) -> ("Triangle out"=w391:T6)
            }
            n118 = for {
              tunnel: w375 -> [w390] mode=indexing
              tunnel: [w389] -> w374 mode=indexing
              workers-P: _ -> [_]
              n119 = call "Process triangle.vi"("Triangle in"=w390) -> ("Triangle out"=w389:T6)
            }
          }
        }
        n120 = case shown="\"Traverse - Tunnel\"" w330 {
          tunnel: ["Collision detection: Traverse - Tunnel" "Collision detection: Traverse - Model" "Collision detection: Traverse - Traverse" "Collision detection: Traverse - Tunnel"] -> w329
          frame "Traverse - Tunnel" {
          }
          frame "Traverse - Model" {
          }
          frame "Traverse - Traverse" {
          }
          frame "Traverse - All", Default {
          }
        }
        n121 = Select(t="Render graphics", s=w342, f="End") -> (s? t:f=w340:string)
        n122 = Select(t=w340, s=w344, f=w329) -> (s? t:f=w343:string)
      }
      frame "Collision detection: Traverse - Tunnel" {
        # "If desired, and no collision, perform minimum separation test within sphere of influence"
        # "Checks traverse triangles against tunnel octrees(and then triangles if necessary)"
        n123 = for {
          workers-P: _ -> [_]
          tunnel: w474 -> [w519] mode=indexing
          tunnel: w440 -> [w518]
          tunnel: w441 -> [w517]
          tunnel: [w515] -> w462 mode=indexing
          tunnel: [w516] -> w453 mode=concatenating if=w515
          tunnel: [w513] -> w452 mode=concatenating if=w512
          n124 = call "Collision test simple.vi"("Octree for query triangles"=w517, "Query triangles"=w518, "Triangle to test"=w519) -> ("Indices of possible triangles"=w513:i32[], "Collision point(s)"=w516:sgl[][], "Collision(s)?"=w515:bool)
          n125 = Empty Array?(array=w513) -> (empty?=w514:bool)
          n126 = Not(x=w514) -> (.not. x?=w512:bool)
        }
        n127 = for {
          workers-P: _ -> [_]
          tunnel: w473 -> [w511] mode=indexing
          tunnel: w440 -> [w510]
          tunnel: w441 -> [w509]
          tunnel: [w507] -> w461 mode=indexing
          tunnel: [w508] -> w455 mode=concatenating if=w507
          tunnel: [w505] -> w451 mode=concatenating if=w504
          n128 = call "Collision test simple.vi"("Octree for query triangles"=w509, "Query triangles"=w510, "Triangle to test"=w511) -> ("Indices of possible triangles"=w505:i32[], "Collision point(s)"=w508:sgl[][], "Collision(s)?"=w507:bool)
          n129 = Empty Array?(array=w505) -> (empty?=w506:bool)
          n130 = Not(x=w506) -> (.not. x?=w504:bool)
        }
        n131 = for {
          workers-P: _ -> [_]
          tunnel: w442 -> [w503] mode=indexing
          tunnel: w440 -> [w502]
          tunnel: w441 -> [w501]
          tunnel: [w499] -> w460 mode=indexing
          tunnel: [w500] -> w454 mode=concatenating if=w499
          tunnel: [w497] -> w450 mode=concatenating if=w496
          n132 = call "Collision test simple.vi"("Octree for query triangles"=w501, "Query triangles"=w502, "Triangle to test"=w503) -> ("Indices of possible triangles"=w497:i32[], "Collision point(s)"=w500:sgl[][], "Collision(s)?"=w499:bool)
          n133 = Empty Array?(array=w497) -> (empty?=w498:bool)
          n134 = Not(x=w498) -> (.not. x?=w496:bool)
        }
        n135 = Or Array Elements(Boolean array=w462) -> (logical OR=w459:bool)
        n136 = Or Array Elements(Boolean array=w461) -> (logical OR=w458:bool)
        n137 = Or Array Elements(Boolean array=w460) -> (logical OR=w457:bool)
        n138 = Build Array(w459, w458, w457) -> (w456:bool[])
        n139 = Build Array (concatenate)(w452, w451, w450) -> (w449:i32[])
        n140 = Or Array Elements(Boolean array=w456) -> (logical OR=w448:bool)
        n141 = call "Remove duplicate indices.vi"("I32 array with duplicates"=w449) -> ("I32 array without duplicates"=w444:i32[])
        n142 = case shown="True" w448 {
          selector: w448 -> [w489 w491]
          tunnel: w455 -> [_ w495]
          tunnel: w454 -> [_ w494]
          tunnel: w453 -> [_ w493]
          tunnel: [sgl[][] [] w492] -> w466
          tunnel: [w489 w491] -> w447
          frame False {
          }
          frame True {
            n143 = Build Array (concatenate)(w493, w495, w494) -> (w492:sgl[][])
          }
        }
        n144 = Compound Arithmetic op=AND(invert w447, w446) -> (w445:bool)
        n145 = case shown="True" w445 {
          tunnel: [sgl 0.0 w487] -> w470
          tunnel: [sgl[] [] w488] -> w469
          tunnel: w444 -> [w479 _]
          tunnel: [w479 w486] -> w443
          tunnel: w442 -> [_ w485]
          tunnel: w439 -> [_ w484]
          tunnel: w441 -> [_ w483]
          tunnel: w440 -> [_ w482]
          frame False {
          }
          frame True {
            n146 = call "Get minimum separation within sphere.vi"("Triangles to test"=w485, "Query triangles"=w482, "Octree for query triangles"=w483, "Sphere of interest"=w484) -> ("Minimum separation vector\n(from all test triangles)"=w488:sgl[], "Minimum separation"=w487:sgl, "Indices of possible triangles"=w486:i32[])  [unwired: 2 in]
          }
        }
        n147 = case shown="\"Traverse - All\"" w465 {
          tunnel: w464 -> [_ w522]
          tunnel: ["Collision detection: Traverse - Model" w521] -> w463
          frame "Traverse - All" {
          }
          frame Default {
            n148 = Select(t="Render graphics", s=w522, f="End") -> (s? t:f=w521:string)
          }
        }
      }
      frame "Collision detection: Traverse - Model" {
        # "append to existing values in case of \"all\" collision mode"
        # "Checks traverse triangles against model octree (and then triangles if necessary)"
        n149 = for {
          workers-P: _ -> [_]
          tunnel: w572 -> [w617] mode=indexing
          tunnel: w531 -> [w616]
          tunnel: w530 -> [w615]
          tunnel: [w613] -> w551 mode=indexing
          tunnel: [w614] -> w546 mode=concatenating if=w613
          tunnel: [w611] -> w543 mode=concatenating if=w610
          n150 = call "Collision test simple.vi"("Octree for query triangles"=w615, "Query triangles"=w616, "Triangle to test"=w617) -> ("Indices of possible triangles"=w611:i32[], "Collision point(s)"=w614:sgl[][], "Collision(s)?"=w613:bool)
          n151 = Empty Array?(array=w611) -> (empty?=w612:bool)
          n152 = Not(x=w612) -> (.not. x?=w610:bool)
        }
        n153 = for {
          workers-P: _ -> [_]
          tunnel: w569 -> [w609] mode=indexing
          tunnel: w531 -> [w608]
          tunnel: w530 -> [w607]
          tunnel: [w605] -> w552 mode=indexing
          tunnel: [w606] -> w545 mode=concatenating if=w605
          tunnel: [w603] -> w542 mode=concatenating if=w602
          n154 = call "Collision test simple.vi"("Octree for query triangles"=w607, "Query triangles"=w608, "Triangle to test"=w609) -> ("Indices of possible triangles"=w603:i32[], "Collision point(s)"=w606:sgl[][], "Collision(s)?"=w605:bool)
          n155 = Empty Array?(array=w603) -> (empty?=w604:bool)
          n156 = Not(x=w604) -> (.not. x?=w602:bool)
        }
        n157 = for {
          workers-P: _ -> [_]
          tunnel: w532 -> [w601] mode=indexing
          tunnel: w531 -> [w600]
          tunnel: w530 -> [w599]
          tunnel: [w597] -> w553 mode=indexing
          tunnel: [w598] -> w544 mode=concatenating if=w597
          tunnel: [w595] -> w541 mode=concatenating if=w594
          n158 = call "Collision test simple.vi"("Octree for query triangles"=w599, "Query triangles"=w600, "Triangle to test"=w601) -> ("Indices of possible triangles"=w595:i32[], "Collision point(s)"=w598:sgl[][], "Collision(s)?"=w597:bool)
          n159 = Empty Array?(array=w595) -> (empty?=w596:bool)
          n160 = Not(x=w596) -> (.not. x?=w594:bool)
        }
        n161 = Or Array Elements(Boolean array=w551) -> (logical OR=w550:bool)
        n162 = Or Array Elements(Boolean array=w552) -> (logical OR=w549:bool)
        n163 = Or Array Elements(Boolean array=w553) -> (logical OR=w548:bool)
        n164 = Build Array(w550, w549, w548) -> (w547:bool[])
        n165 = Build Array (concatenate)(w543, w542, w541) -> (w540:i32[])
        n166 = Or Array Elements(Boolean array=w547) -> (logical OR=w539:bool)
        n167 = case shown="True" w539 {
          selector: w539 -> [w588 w589]
          tunnel: w546 -> [_ w593]
          tunnel: w545 -> [_ w592]
          tunnel: w544 -> [_ w591]
          tunnel: [sgl[][] [] w590] -> w556
          tunnel: [w588 w589] -> w558
          frame False {
          }
          frame True {
            n168 = Build Array (concatenate)(w593, w592, w591) -> (w590:sgl[][])
          }
        }
        n169 = call "Remove duplicate indices.vi"("I32 array with duplicates"=w540) -> ("I32 array without duplicates"=w535:i32[])
        n170 = Or(x=w558, y=w557) -> (x .or. y?=w533:bool)
        n171 = Compound Arithmetic op=AND(invert w533, w529) -> (w538:bool)
        n172 = case shown="True" w538 {
          tunnel: [sgl 0.0 w585] -> w536
          tunnel: [sgl[] [] w586] -> w537
          tunnel: w535 -> [w577 _]
          tunnel: [w577 w584] -> w534
          tunnel: w532 -> [_ w583]
          tunnel: w528 -> [_ w582]
          tunnel: w530 -> [_ w581]
          tunnel: w531 -> [_ w580]
          frame False {
          }
          frame True {
            n173 = call "Get minimum separation within sphere.vi"("Triangles to test"=w583, "Query triangles"=w580, "Octree for query triangles"=w581, "Sphere of interest"=w582) -> ("Minimum separation vector\n(from all test triangles)"=w586:sgl[], "Minimum separation"=w585:sgl, "Indices of possible triangles"=w584:i32[])  [unwired: 2 in]
          }
        }
        n174 = case shown="\"Traverse - All\"" w561 {
          tunnel: w559 -> [_ w620]
          tunnel: ["Collision detection: Traverse - Traverse" w619] -> w560
          frame "Traverse - All" {
          }
          frame Default {
            n175 = Select(t="Render graphics", s=w620, f="End") -> (s? t:f=w619:string)
          }
        }
        n176 = Less?(x=w536, y=w554) -> (x < y?=w565:bool)
        n177 = Build Array (concatenate)(w555, w556) -> (w566:sgl[][])
        n178 = case shown="True" w565 {
          tunnel: w554 -> [w623 _]
          tunnel: w536 -> [_ w625]
          tunnel: [w623 w625] -> w564
          tunnel: w537 -> [_ w626]
          tunnel: [w624 w626] -> w563
          tunnel: w562 -> [w624 _]
          frame False {
          }
          frame True {
          }
        }
      }
      frame "Collision detection: Traverse - Traverse" {
        # "NOT YET IMPLEMENTED!"
        n179 = Select(t="Render graphics", s=w648, f="End") -> (s? t:f=w647:string)
      }
      frame "Render graphics" {
        w660 = T2 {"Red"=0.75, "Green"=0.75, "Blue"=0.75, "Alpha"=1.0} ("Colour")
        w667 = T8."Polygons" ("Render mode")
        n180 = Empty Array?(array=w685) -> (empty?=w684:bool)
        n181 = Not(x=w684) -> (.not. x?=w683:bool)
        n182 = global read "Collision Detection global.vi" "Draw octree leaf-node boxes"() -> (w671:bool)
        n183 = global read "Collision Detection global.vi" "Highlight tested triangles"() -> (w670:bool)
        n184 = And(x=w683, y=w670) -> (x .and. y?=w682:bool)
        n185 = case shown="True" w682 {
          tunnel: w710 -> [w753 w765]
          tunnel: T2 {"Red"=1.0, "Green"=1.0, "Blue"=1.0, "Alpha"=1.0} ("Colour") -> [w752 w766]
          tunnel: w667 -> [w751 w761]
          tunnel: [w750 w755] -> w701
          tunnel: [w748 w760] -> w686
          tunnel: w685 -> [_ w764]
          frame False {
            n186 = call "Create triangles mesh.vi"("Colour"=w752, "Render mode"=w751, "Triangles array"=w753) -> ("Error out"=w750:errorcluster, "Triangle mesh out"=w749:refnum<vi>)
            n187 = Build Array(w749) -> (w748:refnum<vi>[])
          }
          frame True {
            n188 = for {
              tunnel: w765 -> [w775] mode=indexing
              tunnel: w764 -> [w773]
              tunnel: [w775] -> w763 mode=indexing if=w770
              tunnel: [w775] -> w762 mode=indexing if=w774
              shift-right: [w768] -> _
              shift-left: 0 -> [w769]
              i -> [w771]
              n189 = Index Array(array=w773, index=w769) -> (element=w772:i32)
              n190 = Equal?(x=w772, y=w771) -> (x = y?=w770:bool)
              n191 = case shown="True" w770 {
                tunnel: w769 -> [w776 w778]
                tunnel: [w776 w777] -> w768
                frame False {
                }
                frame True {
                  n192 = Increment(x=w778) -> (x+1=w777:i32)
                }
              }
              n193 = Not(x=w770) -> (.not. x?=w774:bool)
            }
            n194 = call "Create triangles mesh.vi"("Colour"=w766, "Render mode"=w761, "Triangles array"=w762) -> ("Error out"=w757:errorcluster, "Triangle mesh out"=w759:refnum<vi>)
            n195 = call "Create triangles mesh.vi"("Colour"=T2 {"Red"=1.0, "Green"=0.85, "Blue"=0.0, "Alpha"=1.0}, "Render mode"=w761, "Triangles array"=w763) -> ("Error out"=w756:errorcluster, "Triangle mesh out"=w758:refnum<vi>)
            n196 = Build Array(w759, w758) -> (w760:refnum<vi>[])
            n197 = Merge Errors(w757, w756) -> (w755:errorcluster)
          }
        }
        n198 = Empty Array?(array=w664) -> (empty?=w680:bool)
        n199 = Not(x=w680) -> (.not. x?=w681:bool)
        n200 = And(x=w681, y=w670) -> (x .and. y?=w663:bool)
        n201 = case shown="True" w663 {
          tunnel: w666 -> [w722 w734]
          tunnel: T2 {"Red"=0.5, "Green"=0.5, "Blue"=0.5, "Alpha"=1.0} ("Colour") -> [w721 w735]
          tunnel: w667 -> [w720 w730]
          tunnel: [w719 w724] -> w662
          tunnel: [w717 w729] -> w665
          tunnel: w664 -> [_ w733]
          frame False {
            n202 = call "Create triangles mesh.vi"("Colour"=w721, "Render mode"=w720, "Triangles array"=w722) -> ("Error out"=w719:errorcluster, "Triangle mesh out"=w718:refnum<vi>)
            n203 = Build Array(w718) -> (w717:refnum<vi>[])
          }
          frame True {
            n204 = for {
              tunnel: w734 -> [w744] mode=indexing
              tunnel: w733 -> [w742]
              tunnel: [w744] -> w732 mode=indexing if=w739
              tunnel: [w744] -> w731 mode=indexing if=w743
              shift-right: [w737] -> _
              shift-left: 0 -> [w738]
              i -> [w740]
              n205 = Index Array(array=w742, index=w738) -> (element=w741:i32)
              n206 = Equal?(x=w741, y=w740) -> (x = y?=w739:bool)
              n207 = case shown="True" w739 {
                tunnel: w738 -> [w745 w747]
                tunnel: [w745 w746] -> w737
                frame False {
                }
                frame True {
                  n208 = Increment(x=w747) -> (x+1=w746:i32)
                }
              }
              n209 = Not(x=w739) -> (.not. x?=w743:bool)
            }
            n210 = call "Create triangles mesh.vi"("Colour"=w735, "Render mode"=w730, "Triangles array"=w731) -> ("Error out"=w726:errorcluster, "Triangle mesh out"=w728:refnum<vi>)
            n211 = call "Create triangles mesh.vi"("Colour"=T2 {"Red"=1.0, "Green"=0.85, "Blue"=0.0, "Alpha"=1.0}, "Render mode"=w730, "Triangles array"=w732) -> ("Error out"=w725:errorcluster, "Triangle mesh out"=w727:refnum<vi>)
            n212 = Build Array(w728, w727) -> (w729:refnum<vi>[])
            n213 = Merge Errors(w726, w725) -> (w724:errorcluster)
          }
        }
        n214 = call "Create triangles mesh.vi"("Colour"=w660, "Render mode"=w667, "Triangles array"=w709) -> ("Error out"=w700:errorcluster, "Triangle mesh out"=w692:refnum<vi>)
        n215 = call "Create triangles mesh.vi"("Colour"=w660, "Render mode"=w667, "Triangles array"=w708) -> ("Error out"=w699:errorcluster, "Triangle mesh out"=w691:refnum<vi>)
        n216 = call "Create triangles mesh.vi"("Colour"=w660, "Render mode"=w667, "Triangles array"=w707) -> ("Error out"=w698:errorcluster, "Triangle mesh out"=w690:refnum<vi>)
        n217 = Build Array (concatenate)(w686, w665, w692, w691, w690) -> (w678:refnum<vi>[])
        n218 = case shown="True" w671 {
          tunnel: w706 -> [_ w803]
          tunnel: w705 -> [_ w802]
          tunnel: T2 {"Red"=0.0, "Green"=0.25, "Blue"=0.0, "Alpha"=1.0} ("Colour (emission)") -> [_ w799]
          tunnel: T2 {"Red"=0.0, "Green"=0.5, "Blue"=0.5, "Alpha"=1.0} ("Colour (emission)") -> [_ w798]
          tunnel: [errorcluster {"status"=FALSE, "code"=0, "source"=""} ("error IO") w792] -> w697
          tunnel: [w790 w791] -> w677
          tunnel: w678 -> [w790 w795]
          frame False {
          }
          frame True {
            n219 = call "Create Octree node boxes.vi"("Colour (emission)"=w799, "Draw populated leaf nodes only"=TRUE, "Octree nodes array"=w803) -> ("Error out"=w794:errorcluster, "Octree node boxes array"=w797:refnum<vi>[])
            n220 = call "Create Octree node boxes.vi"("Colour (emission)"=w798, "Draw populated leaf nodes only"=TRUE, "Octree nodes array"=w802) -> ("Error out"=w793:errorcluster, "Octree node boxes array"=w796:refnum<vi>[])
            n221 = Build Array (concatenate)(w795, w797, w796) -> (w791:refnum<vi>[])
            n222 = Merge Errors(w794, w793) -> (w792:errorcluster)
          }
        }
        n223 = global read "Collision Detection global.vi" "Collision marker radius (mm)"() -> (w669:sgl)
        n224 = Empty Array?(array=w658) -> (empty?=w687:bool)
        n225 = case shown="False" w687 {
          tunnel: T3 {"Red"=1.0, "Green"=0.0, "Blue"=0.0, "Alpha"=1.0} ("Colour") -> [w786 _]
          tunnel: w669 -> [w785 _]
          tunnel: w667 -> [w784 _]
          tunnel: [w783 errorcluster {"status"=FALSE, "code"=0, "source"=""} ("error IO")] -> w696
          tunnel: [w781 w788] -> w676
          tunnel: w677 -> [w782 w788]
          tunnel: w658 -> [w779 _]
          frame False {
            n226 = call "Create spheres.vi"("Render mode"=w784, "Colour"=w786, "Radius (model units)"=w785, "Points array"=w779) -> ("Error out"=w783:errorcluster, "Points"=w780:refnum<vi>[])
            n227 = Build Array (concatenate)(w782, w780) -> (w781:refnum<vi>[])
          }
          frame True {
          }
        }
        n228 = global read "Collision Detection global.vi" "Camera Position"() -> (w674:T9)
        n229 = global read "Collision Detection global.vi" "Reset camera"() -> (w659:bool)
        n230 = global read "Collision Detection global.vi" "Up Direction"() -> (w672:T9)
        n231 = global read "Collision Detection global.vi" "Target"() -> (w673:T9)
        n232 = call "Create new scene.vi"("Translation"=cluster{"X":sgl, "Y":sgl, "Z":sgl} {"X"=0.0, "Y"=0.0, "Z"=0.0}, "Scale"=cluster{"X":sgl, "Y":sgl, "Z":sgl} {"X"=1.0, "Y"=1.0, "Z"=1.0}, "Scene objects array"=w676) -> ("Error out"=w695:errorcluster, "Scene out"=w679:refnum<vi>)
        n233 = call "3D display.vi"("Camera Position"=w674, "Scene in"=w679, "Target"=w673, "Up Direction"=w672, "Reset camera"=w659) -> ()  [unwired: 1 in]
        n234 = Merge Errors(w694, w701, w662, w700, w699, w698, w697, w696, w695) -> (w693:errorcluster)
      }
      frame "End" {
        n235 = case shown="True" w813 {
          tunnel: w812 -> [_ w836]
          tunnel: w811 -> [_ w835]
          tunnel: w810 -> [_ w834]
          tunnel: [w833 w836] -> w809
          tunnel: [w832 w835] -> w808
          tunnel: [w831 w834] -> w807
          tunnel: w806 -> [w831 _]
          tunnel: w805 -> [w832 _]
          tunnel: w804 -> [w833 _]
          frame False {
          }
          frame True {
          }
        }
      }
    }
  }
  "Collision" <- w16
  "Minimum separation" <- w15
  "Minimum separation vector (from trav.)" <- w14
  "Collision point(s)" <- w13
  "Error out" <- w12
